vi "Setup.vi"(11 "Setup in":refnum<class "Setup.lvclass">) -> (3 "Setup out":refnum<class "Setup.lvclass">)   [LabVIEW 2021, in "jettl.lvlib" / "Setup.lvlib" / "Setup.lvclass"]
uses:
  Setup.lvclass
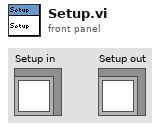
[diagram p1: front panel]
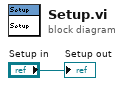
[diagram p0: block diagram]
diagram:
  "Setup out" <- "Setup in"
